vi "xcorrectionLUT_coMD.vi"() -> ()   [LabVIEW 2012]
doc: "SciScan 1.2 160622"
uses:
  <vilib>/Utility/VariantDataType/Type.ctl
  GFG/GFGfpRefGet.vi
  GFG/GFG library.lvlib
  <vilib>/Utility/VariantDataType/VariantType.lvlib
panel:
  out "error out 2":errorcluster
  out "error out":errorcluster
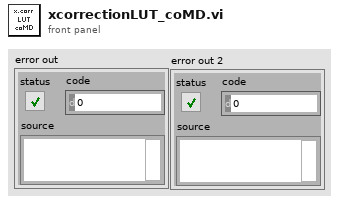
[diagram p1: front panel]
types:
  T1 = cluster{"WaveformChartRef":refnum<vi>, "DigitalRef":refnum<vi>, "ArrayRef":refnum<vi>, "TabControlRef":refnum<vi>, "EnumRef":refnum<vi>, "RingRef":refnum<vi>, "BooleanRef":refnum<vi>, "KnobRef":refnum<vi>, "SlideRef":refnum<vi>, "PathRef":refnum<vi>, "StringRef":refnum<vi>, "ComboBox":refnum<vi>, "WaveformGraphRef":refnum<vi>}
  T2 = enum16{"open", "replace", "create", "open or create", "replace or create", "replace or create with confirmation"}
  T3 = cluster{cluster{"[0]":variant, "[1]":variant, "[2]":variant}[], variant[]}
  T4 = cluster{"[0]":variant, "[1]":variant, "[2]":variant}
  T5 = cluster{"[0]":variant, "[1]":variant, "[2]":variant}[]
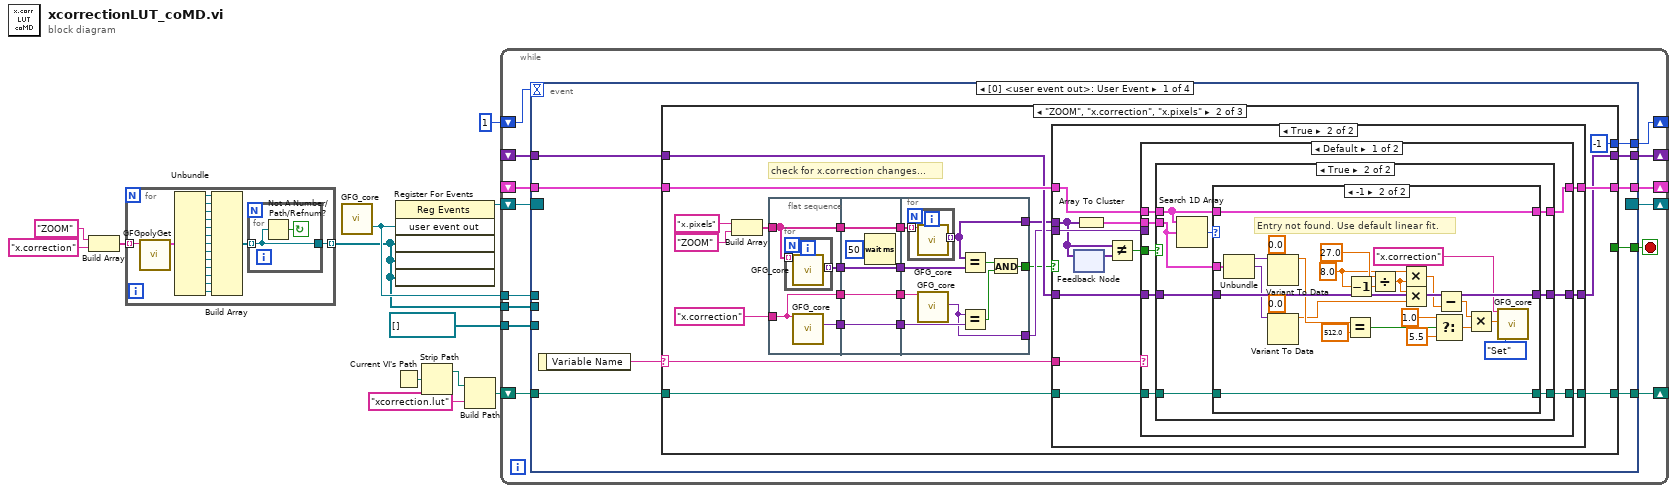
[diagram p0: block diagram]
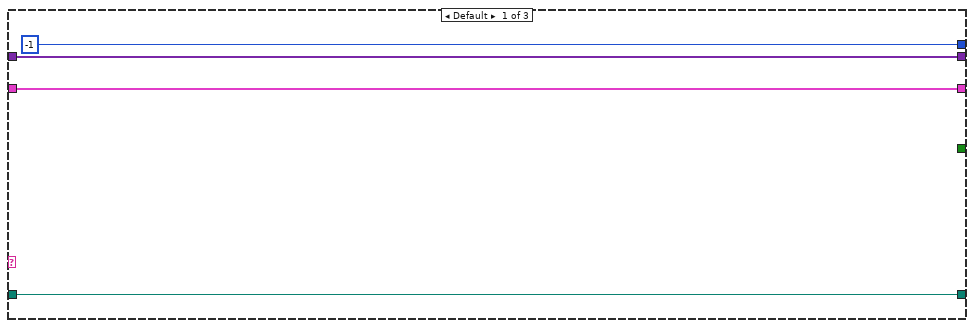
[diagram p2: hidden frame]
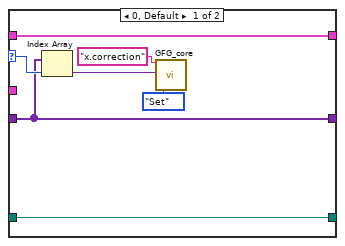
[diagram p5: hidden frame]
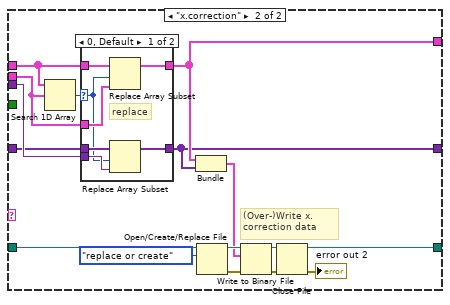
[diagram p6: hidden frame]
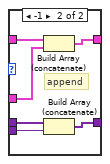
[diagram p7: hidden frame]
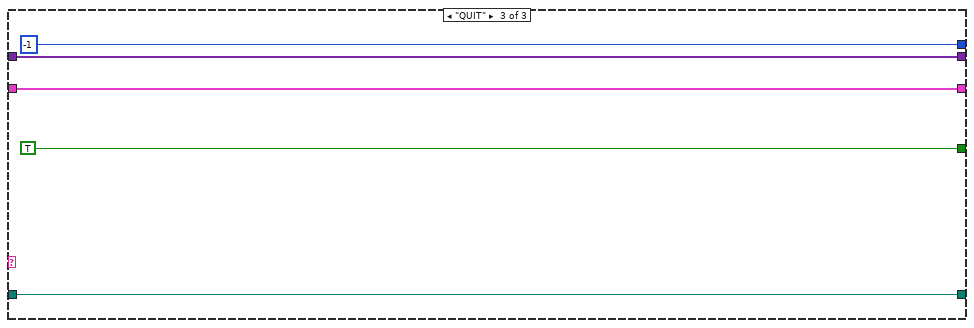
[diagram p8: hidden frame]
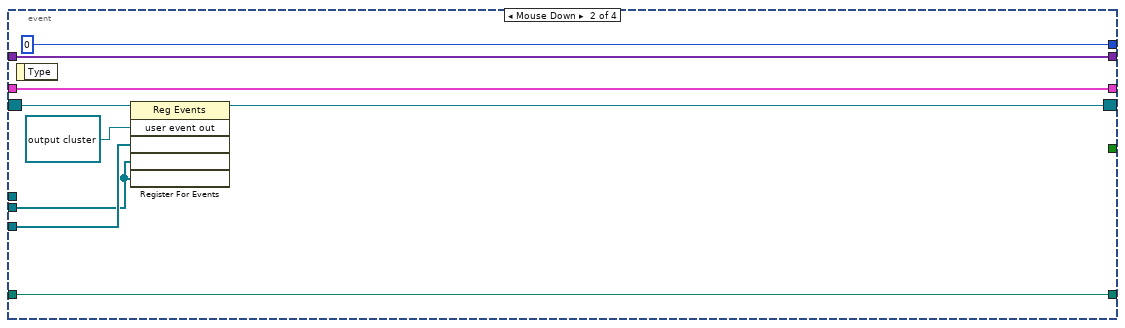
[diagram p9: hidden frame]
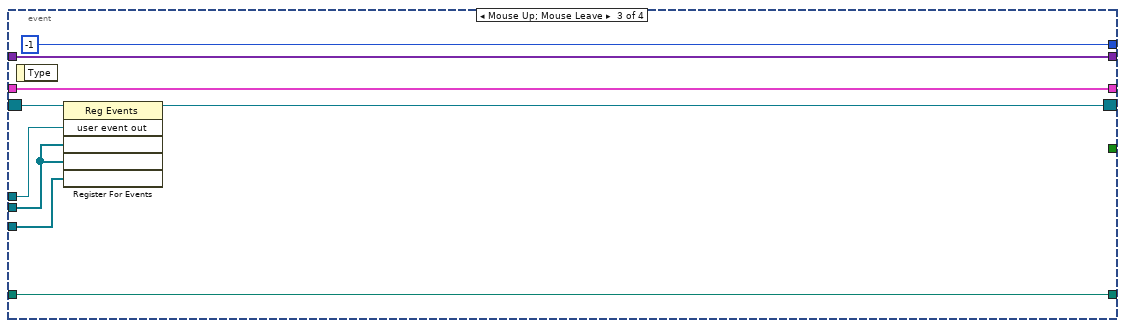
[diagram p10: hidden frame]
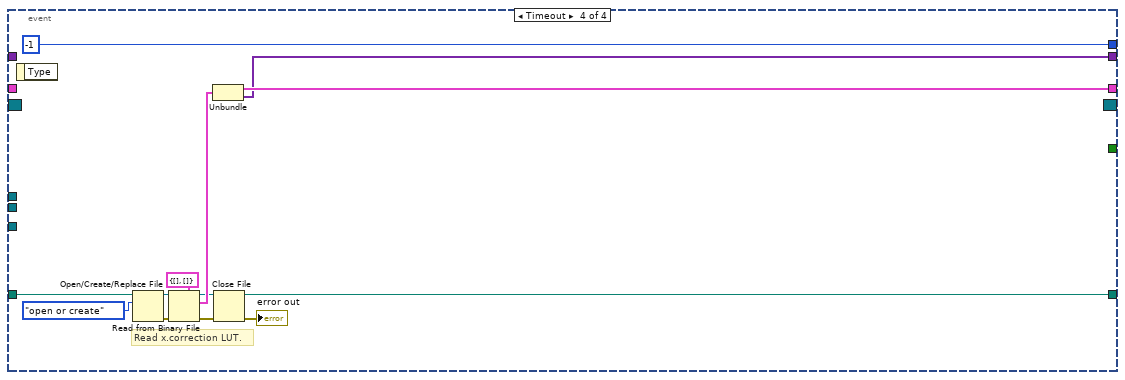
[diagram p11: hidden frame]
diagram:
  n1 = Build Array("ZOOM", "x.correction") -> (w8:string[])
  n2 = for {
    tunnel: w8 -> [w29] mode=indexing
    tunnel: [w13] -> w4 mode=indexing
    n3 = call-poly "GFGpolyGet.vi"("Variable Name in"=w29) -> ("output cluster"=w15:T1)  [unwired: 9 in, 1 out]
    n4 = Unbundle(w15) -> ("WaveformChartRef"=w26:refnum<vi>, "DigitalRef"=w25:refnum<vi>, "ArrayRef"=w24:refnum<vi>, "TabControlRef"=w23:refnum<vi>, "EnumRef"=w22:refnum<vi>, "RingRef"=w21:refnum<vi>, "BooleanRef"=w20:refnum<vi>, "KnobRef"=w19:refnum<vi>, "SlideRef"=w18:refnum<vi>, "PathRef"=w17:refnum<vi>, "StringRef"=w16:refnum<vi>, "ComboBox"=w27:refnum<vi>, "WaveformGraphRef"=w28:refnum<vi>)
    n5 = Build Array(w26, w25, w24, w23, w22, w21, w20, w19, w18, w17, w16, w27, w28) -> (w14:refnum<vi>[])
    n6 = for {
      tunnel: w14 -> [w30] mode=indexing
      tunnel: [w30] -> w13
      stop <- w31 continue-if-true
      n7 = Not A Number/Path/Refnum?(number/path/refnum=w30) -> (NaN/Path/Refnum?=w31:bool)
    }
  }
  n8 = call "GFG_core.vi"() -> ("user event out"=w5:refnum<user-event>)  [unwired: 13 in, 6 out]
  n9 = Current VI's Path() -> (path=w11:path)
  n10 = register-events(w5, w4, w4, w4) -> (reference out=w12:refnum<event-registration>)  [unwired: 2 in, 1 out]
  n11 = Strip Path(path=w11) -> (stripped path=w2:path)  [unwired: 1 out]
  n12 = Build Path(base path=w2, name or relative path="xcorrection.lut") -> (appended path=w10:path)
  n13 = while {
    shift-right: [w41] -> _
    shift-left: _ -> [w42]
    shift-right: [w39] -> _
    shift-left: _ -> [w40]
    shift-right: [w38] -> _
    shift-left: 1 -> [w37]
    tunnel: w4 -> [w36]
    shift-right: [w35] -> _
    shift-left: w12 -> [w45]
    tunnel: w5 -> [w34]
    tunnel: refnum<vi>[] [] ("event source") -> [w33]
    shift-right: [w32] -> _
    shift-left: w10 -> [w44]
    stop <- w43 stop-if-true
    n14 = event shown="[0] <user event out>: User Event" {
      selector: w45 -> [_ w212 w221 _]
      dyn-events: [_ w210 w220 _] -> w35
      timeout: w37 -> [_ _ _ _]
      tunnel: w44 -> [w53 w207 w216 w225]
      tunnel: [w52 _ _ _] -> w43
      tunnel: w42 -> [w51 w205 w213 _]
      tunnel: [w50 w205 w213 w224] -> w41
      tunnel: w40 -> [w49 w204 w215 _]
      tunnel: [w48 w204 w215 w223] -> w39
      tunnel: [w46 0 -1 -1] -> w38
      tunnel: w36 -> [_ w208 w218 _]
      tunnel: w34 -> [_ _ w219 _]
      tunnel: w33 -> [_ w209 w217 _]
      tunnel: [w47 w207 w216 w222] -> w32
      event User Event {
        n15 = event-data() -> ("Variable Name"=w54:string)  [unwired: 1 in]
        n16 = case shown="\"ZOOM\", \"x.correction\", \"x.pixels\"" w54 {
          selector: w54 -> [_ w77 _]
          tunnel: w53 -> [w56 w75 w200]
          tunnel: [_ _ TRUE] -> w52
          tunnel: w51 -> [w57 w81 w201]
          tunnel: [w57 w80 w201] -> w50
          tunnel: w49 -> [w58 w79 w202]
          tunnel: [w58 w78 w202] -> w48
          tunnel: [w56 w74 w200] -> w47
          tunnel: [-1 -1 -1] -> w46
          frame Default {
          }
          frame "ZOOM", "x.correction", "x.pixels" {
            # "check for x.correction changes..."
            n17 = Build Array("x.pixels", "ZOOM") -> (w64:string[])
            n18 = flat-sequence {
              tunnel: w64 -> [w85]
              tunnel: [w85] -> w73
              tunnel: [w84] -> w72
              tunnel: "x.correction" -> [w83]
              tunnel: [w83] -> w71
              tunnel: [w82] -> w70
              tunnel: [w91] -> w69
              tunnel: w73 -> [w91]
              tunnel: [w90] -> w68
              tunnel: w72 -> [w90]
              tunnel: [w89] -> w67
              tunnel: w71 -> [w89]
              tunnel: w70 -> [w88]
              tunnel: [w88] -> w66
              tunnel: [w96] -> w59
              tunnel: w69 -> [w100]
              tunnel: w68 -> [w99]
              tunnel: w67 -> [w98]
              tunnel: w66 -> [w97]
              tunnel: [w94] -> w60
              tunnel: [w93] -> w61
              frame #0 {
                n19 = for {
                  tunnel: w85 -> [w87] mode=indexing
                  tunnel: [w86] -> w84 mode=indexing
                  n20 = call "GFG_core.vi"("Variable Name in"=w87) -> ("Variant Out"=w86:variant)  [unwired: 12 in, 6 out]
                }
                n21 = call "GFG_core.vi"("Variable Name in"=w83) -> ("Variant Out"=w82:variant)  [unwired: 12 in, 6 out]
              }
              frame #1 {
                n22 = Wait (ms)(milliseconds to wait=u32 50) -> ()  [unwired: 1 out]
              }
              frame #2 {
                n23 = for {
                  tunnel: [w103] -> w93 mode=indexing
                  tunnel: w100 -> [w102] mode=indexing
                  n24 = call "GFG_core.vi"("Variable Name in"=w102) -> ("Variant Out"=w103:variant)  [unwired: 12 in, 6 out]
                }
                n25 = call "GFG_core.vi"("Variable Name in"=w98) -> ("Variant Out"=w94:variant)  [unwired: 12 in, 6 out]
                n26 = Equal?(x=w93, y=w99) -> (x = y?=w101:bool)
                n27 = Equal?(x=w94, y=w97) -> (x = y?=w95:bool)
                n28 = And(x=w101, y=w95) -> (x .and. y?=w96:bool)
              }
            }
            n29 = case shown="True" w59 {
              tunnel: w75 -> [w104 w117]
              tunnel: w81 -> [w106 w115]
              tunnel: [w106 w114] -> w80
              tunnel: w79 -> [w105 w113]
              tunnel: [w105 w112] -> w78
              tunnel: w77 -> [_ w111]
              tunnel: w60 -> [_ w109]
              tunnel: w61 -> [_ w107]
              tunnel: [w104 w108] -> w74
              frame False {
              }
              frame True {
                n30 = feedback #1() -> (w116:variant[])  [unwired: 1 in]
                n31 = feedback-in #1(w107) -> ()
                n32 = Array To Cluster(array=w107) -> (cluster=w118:T4)
                n33 = Not Equal?(x=w107, y=w116) -> (x != y?=w110:bool)
                n34 = case shown="Default" w111 {
                  tunnel: w118 -> [w126 w182]
                  tunnel: w115 -> [w124 w185]
                  tunnel: w109 -> [_ w184]
                  tunnel: [w123 w181] -> w114
                  tunnel: w113 -> [w125 w183]
                  tunnel: w117 -> [w120 w179]
                  tunnel: [w122 w180] -> w112
                  tunnel: w110 -> [w121 _]
                  tunnel: [w119 w178] -> w108
                  frame Default {
                    n35 = case shown="True" w121 {
                      tunnel: w126 -> [_ w130]
                      tunnel: w125 -> [w128 w136]
                      tunnel: w124 -> [w129 w135]
                      tunnel: [w129 w134] -> w123
                      tunnel: [w128 w133] -> w122
                      tunnel: w120 -> [w127 w132]
                      tunnel: [w127 w131] -> w119
                      frame False {
                      }
                      frame True {
                        n36 = Search 1D Array(1D array=w135, element=w130) -> (index of element=w137:i32)  [unwired: 1 in]
                        n37 = case shown="-1" w137 {
                          selector: w137 -> [w143 _]
                          tunnel: w135 -> [w144 w169]
                          tunnel: [w144 w169] -> w134
                          tunnel: w136 -> [w142 w168]
                          tunnel: [w142 w168] -> w133
                          tunnel: w132 -> [w138 w167]
                          tunnel: [w138 w167] -> w131
                          tunnel: w130 -> [_ w166]
                          frame 0, Default {
                            n38 = Index Array(array=w142, index=w143) -> (element=w139:variant)
                            n39 = call "GFG_core.vi"("Variable Name in"="x.correction", "Variant in"=w139, "Action"=enum16{"Init", "Set", "Get", "Clear"}."Set") -> ()  [unwired: 10 in, 7 out]
                          }
                          frame -1 {
                            w158 = 8.0
                            # "Entry not found. Use default linear fit."
                            n40 = Unbundle(w166) -> ("[0]"=w164:variant, "[1]"=w163:variant)  [unwired: 1 out]
                            n41 = Variant To Data(type=0.0, Variant=w164) -> (data=w147:dbl)  [unwired: 1 in, 1 out]
                            n42 = Variant To Data(type=0.0, Variant=w163) -> (data=w146:dbl)  [unwired: 1 in, 1 out]
                            n43 = Equal?(x=w147, y=512.0) -> (x = y?=w149:bool)
                            n44 = Decrement(x=w158) -> (x-1=w157:dbl)
                            n45 = Divide(x=27.0, y=w157) -> (x/y=w156:dbl)
                            n46 = Multiply(x=w158, y=w156) -> (x*y=w154:dbl)
                            n47 = Multiply(x=w156, y=w146) -> (x*y=w153:dbl)
                            n48 = Select(t=1.0, s=w149, f=5.5) -> (s? t:f=w152:dbl)
                            n49 = Subtract(x=w153, y=w154) -> (x-y=w155:dbl)
                            n50 = Multiply(x=w155, y=w152) -> (x*y=w162:dbl)
                            n51 = call "GFG_core.vi"("Variable Name in"="x.correction", "Variant in"=w162, "Action"=enum16{"Init", "Set", "Get", "Clear"}."Set") -> ()  [unwired: 10 in, 7 out]
                          }
                        }
                      }
                    }
                  }
                  frame "x.correction" {
                    # "(Over-)Write x.correction data"
                    n52 = Search 1D Array(1D array=w185, element=w182) -> (index of element=w177:i32)  [unwired: 1 in]
                    n53 = case shown="0, Default" w177 {
                      selector: w177 -> [w187 _]
                      tunnel: w185 -> [w192 w198]
                      tunnel: w182 -> [w191 w197]
                      tunnel: [w190 w196] -> w181
                      tunnel: w183 -> [w189 w195]
                      tunnel: w184 -> [w188 w193]
                      tunnel: [w186 w194] -> w180
                      frame 0, Default {
                        # "replace"
                        n54 = Replace Array Subset(array=w192, new element=w191, index=w187) -> (w190:T5)
                        n55 = Replace Array Subset(array=w189, new element=w188, index=w187) -> (w186:variant[])
                      }
                      frame -1 {
                        # "append"
                        n56 = Build Array (concatenate)(w198, w197) -> (w196:T5)
                        n57 = Build Array (concatenate)(w195, w193) -> (w194:variant[])
                      }
                    }
                    n58 = Bundle(w181, w180) -> (w171:T3)  [unwired: 1 in]
                    n59 = Open/Create/Replace File(file path (use dialog)=w179, operation (0:open)=T2."replace or create") -> (refnum out=w176:refnum<file>, error out=w173:errorcluster)  [unwired: 4 in, 1 out]
                    n60 = Write to Binary File(file (use dialog)=w176, data=w171, error in=w173) -> (refnum out=w175:refnum<file>, error out=w174:errorcluster)  [unwired: 3 in, 1 out]
                    n61 = Close File(refnum=w175, error in=w174) -> (path=w178:path, error out=→"error out 2":errorcluster)
                  }
                }
              }
            }
          }
          frame "QUIT" {
          }
        }
      }
      event Mouse Down {
        n62 = event-data() -> ()  [unwired: 1 in, 1 out]
        n63 = register-events(reference=w212, refnum<user-event> refnum ("user event out"), w209, w208, w208) -> (reference out=w210:refnum<event-registration>)  [unwired: 1 in, 1 out]
      }
      event Mouse Up; Mouse Leave {
        n64 = event-data() -> ()  [unwired: 1 in, 1 out]
        n65 = register-events(reference=w221, w219, w218, w218, w217) -> (reference out=w220:refnum<event-registration>)  [unwired: 1 in, 1 out]
      }
      event Timeout {
        # "Read x.correction LUT."
        n66 = event-data() -> ()  [unwired: 1 in, 1 out]
        n67 = Open/Create/Replace File(file path (use dialog)=w225, operation (0:open)=T2."open or create") -> (refnum out=w232:refnum<file>, error out=w228:errorcluster)  [unwired: 4 in, 1 out]
        n68 = Read from Binary File(5:T3 {[], []} ("output cluster"), 8:w228, 11:w232) -> (0:w229:errorcluster, 2:w233:T3, 3:w230:refnum<file>)  [unwired: 3 in, 1 out]
        n69 = Unbundle(w233) -> (w224:T5, w223:variant[])
        n70 = Close File(refnum=w230, error in=w229) -> (path=w222:path, error out=→"error out":errorcluster)
      }
    }
  }
